vi "Configure Data Log Measurement Range.vi"(6 "Data Log Auto Range (False)":bool, 7 "Data Log Measurement Range (0.0)":dbl format="%^.3e", 8 "error in (no error)":errorcluster {"code" format="%.0x"}, 9 "Data Log Type (1: Voltage)":i32(ring)=1 items=["Voltage"=1, "Current"=0], 10 "Channel Name (1)":string="1", 11 "VISA resource name":refnum<visa-resource-name>) -> (0 "error out":errorcluster {"code" format="%.0x"}, 3 "VISA resource name out":refnum<visa-resource-name>)   [LabVIEW 2018, in "Agilent N6700 Series.lvlib"]
doc: "Configures the measurement range of the data logger.\n\n<b>Note:</b>\nThis VI only applies to the N6705B and N6705C DC Power Analyzer."
uses:
  Agilent N6700 Series.lvlib
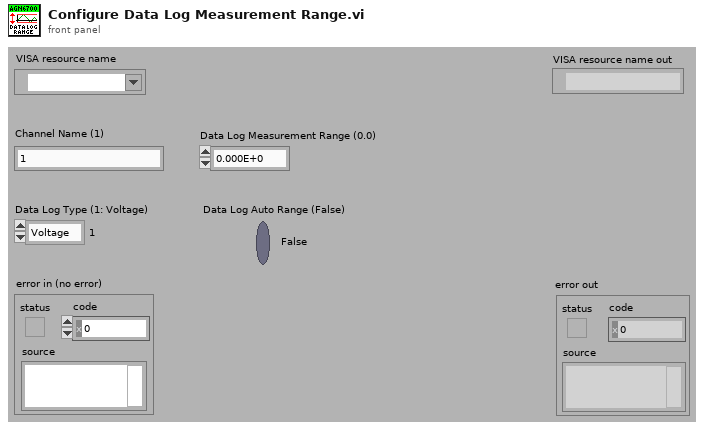
[diagram p1: front panel]
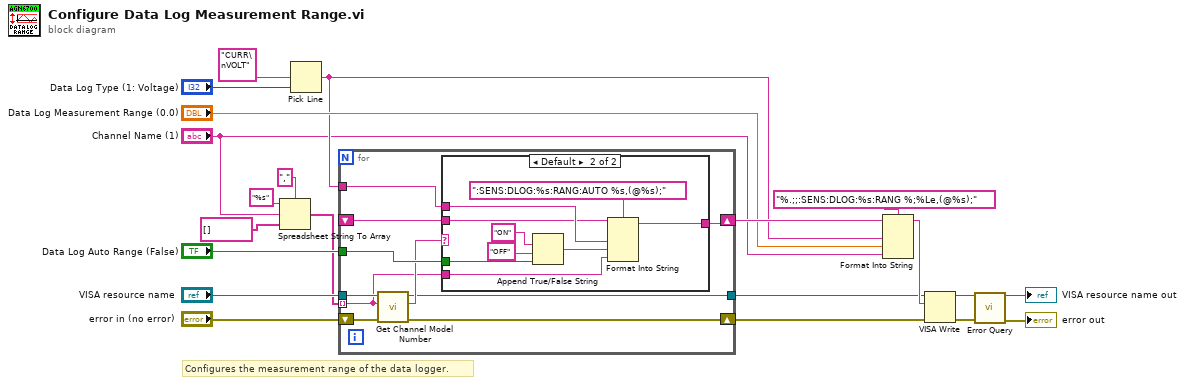
[diagram p0: block diagram]
diagram:
  # "Configures the measurement range of the data logger."
  n1 = Spreadsheet String To Array(delimiter (Tab)=",", format string="%s", spreadsheet string="Channel Name (1)", array type (2D Dbl)=string[] []) -> (array=w1:string[])
  n2 = Pick Line(multi-line string="CURR\nVOLT", line index="Data Log Type (1: Voltage)") -> (output string=w6:string)  [unwired: 1 in]
  n3 = for {
    tunnel: "Data Log Auto Range (False)" -> [w30]
    shift-right: [w31] -> w17
    shift-left: _ -> [w22]
    tunnel: w1 -> [w25] mode=indexing
    tunnel: "VISA resource name" -> [w29]
    shift-right: [w27] -> w8
    shift-left: "error in (no error)" -> [w28]
    tunnel: [w24] -> w7
    tunnel: w6 -> [w23]
    n4 = call "Get Channel Model Number.vi"("error in (no error)"=w28, "Channel Name (1)"=w25, "VISA resource name"=w29) -> ("error out"=w27:errorcluster, "Model Number"=w26:string, "VISA resource name out"=w24:refnum<visa-resource-name>)  [unwired: 6 in]
    n5 = case shown="Default" w26 {
      tunnel: [w32 w41] -> w31
      tunnel: w23 -> [w32 w40]
      tunnel: w30 -> [_ w35]
      tunnel: w25 -> [_ w34]
      tunnel: w22 -> [_ w33]
      frame "N6791A", "N6792A" {
        # "N679x models doesn't support AUTO Range"
      }
      frame Default {
        n6 = Append True/False String(1:w35, 2:"OFF", 3:"ON") -> (0:w36:string)  [unwired: 1 in]
        n7 = Format Into String(format string=":SENS:DLOG:%s:RANG:AUTO %s,(@%s);", initial string=w33, w40, w36, w34) -> (resulting string=w41:string)  [unwired: 1 in, 1 out]
      }
    }
  }
  n8 = Format Into String(format string="%.;;:SENS:DLOG:%s:RANG %;%Le,(@%s);", initial string=w17, w6, "Data Log Measurement Range (0.0)", "Channel Name (1)") -> (resulting string=w16:string)  [unwired: 1 in, 1 out]
  n9 = VISA Write(VISA resource name=w7, write buffer=w16, error in (no error)=w8) -> (VISA resource name out=w19:refnum<visa-resource-name>, error out=w18:errorcluster)  [unwired: 1 out]
  n10 = call "Error Query.vi"("VISA resource name"=w19, "error in (no error)"=w18) -> ("VISA resource name out"=→"VISA resource name out":refnum<visa-resource-name>, "error out"=→"error out":errorcluster)  [unwired: 10 in, 2 out]
